vi "mxwScript_API_XML_DeuniquifyOnly.vi"(8 "error in (no error)":errorcluster, 10 "deuniquifyOnly?":bool=TRUE, 11 "control name":string) -> (0 "error out":errorcluster, 3 "encoded control name":string)   [LabVIEW 2020]
doc: "Add diagram to drop this template into to the template name."
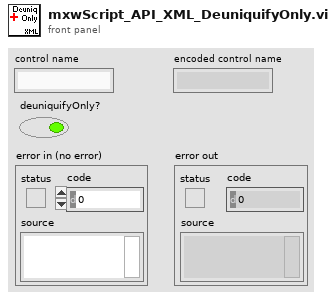
[diagram p1: front panel]
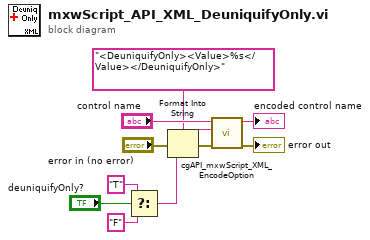
[diagram p0: block diagram]
diagram:
  n1 = Select(t="T" ("input 1"), s="deuniquifyOnly?", f="F" ("input 1")) -> (s? t:f=w3:string)
  n2 = Format Into String(format string="<DeuniquifyOnly><Value>%s</Value></DeuniquifyOnly>" ("control name"), error in="error in (no error)", w3) -> (resulting string=w6:string, error out=w8:errorcluster)  [unwired: 1 in]
  n3 = call "cgAPI_mxwScript_XML_EncodeOption.vi"("error in (no error)"=w8, "otherXML"=w6, "normalTextString"="control name") -> ("error out"=→"error out":errorcluster, "encodedString"=→"encoded control name":string)  [unwired: 7 out]
